vi "Get Spectrum.vi"(8 "error in (no error)":errorcluster, 10 "Channel":u8, 11 "Ocean Optics Driver in":refnum<class "Ocean Optics Driver.lvclass">) -> (0 "error out":errorcluster, 2 "Spectrum Graph":T1(graph), 3 "Ocean Optics Driver out":refnum<class "Ocean Optics Driver.lvclass">)   [LabVIEW 2016, in "Ocean Optics Driver.lvclass"]
uses:
  Ocean Optics Driver.lvclass
  <instrlib>/Ocean Optics 2000 4000/Ocean Optics 2000 4000.lvlib
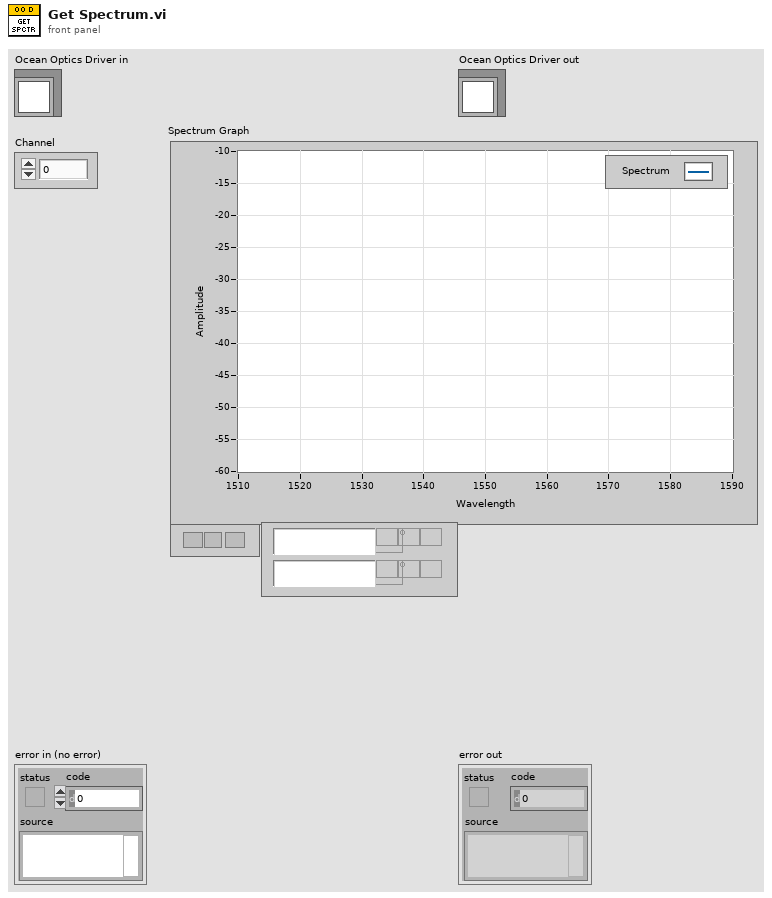
[diagram p1: front panel]
types:
  T1 = cluster{"Wavelengths":dbl[], "Spectrum by Pixel Number":dbl[]}[]
  T2 = typedef "Ocean optics configuration.ctl" = cluster{"Integration time":dbl, "Fit parameters":T3, "Fit":bool, "Auto-update params":bool, "Save spectra":bool}
  T3 = typedef "Multi-peak Parameters.ctl" = cluster{"Peaks":T4[], "Function":enum16{"Gauss", "Lorentz"}, "Window width":dbl}
  T4 = typedef "Peak Parameters.ctl" = cluster{"Amplitude":dbl, "Center":dbl, "Width":dbl}
  T5 = cluster{"Accessors:Wavelengths":dbl[], "Spectrum by Pixel Number":dbl[]}
  T6 = cluster{"Accessors:Wavelengths":dbl[], "Spectrum by Pixel Number":dbl[]}[]
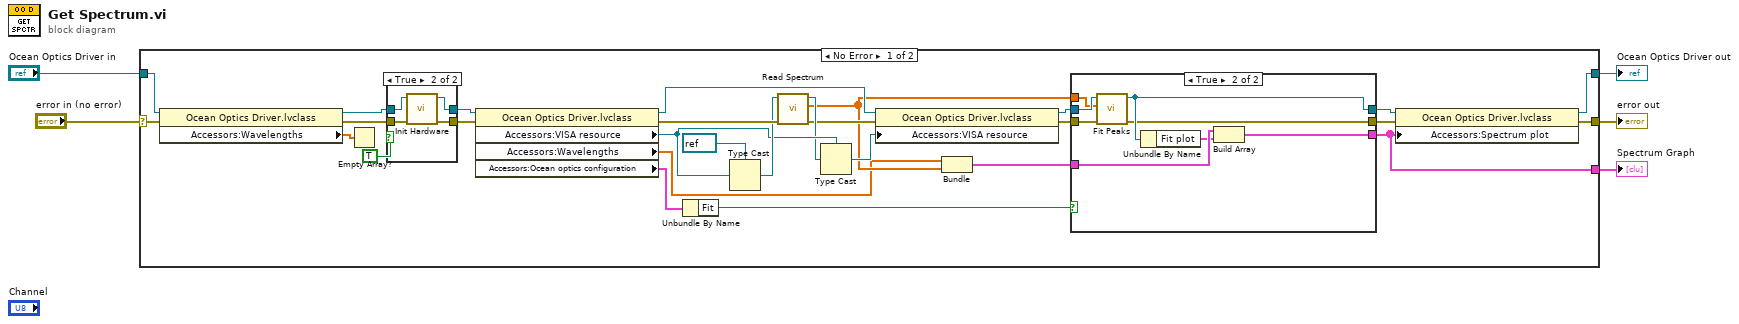
[diagram p0: block diagram]
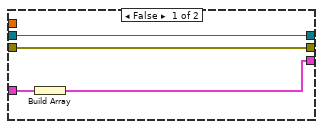
[diagram p3: hidden frame]
diagram:
  n1 = case shown="No Error" "error in (no error)" {
    selector: "error in (no error)" -> [w14 w52]
    tunnel: "Ocean Optics Driver in" -> [w12 w53]
    tunnel: [w18 w52] -> w4
    tunnel: [w16 w53] -> w3
    tunnel: [w15 _] -> w2
    frame No Error {
      n2 = property class="Ocean Optics Driver.lvclass"(reference=w12, error in=w14) -> (reference out=w10:refnum<class "Ocean Optics Driver.lvclass">, error out=w9:errorcluster, "Accessors:Wavelengths"=w11:dbl[])
      n3 = Empty Array?(array=w11) -> ()  [unwired: 1 out]
      n4 = case shown="True" TRUE {
        tunnel: w10 -> [w35 w39]
        tunnel: w9 -> [w34 w38]
        tunnel: [w35 w37] -> w8
        tunnel: [w34 w36] -> w7
        frame False {
        }
        frame True {
          n5 = call-dynamic "Init Hardware.vi"("error in (no error)"=w38, "Ocean Optics Driver in"=w39) -> ("error out"=w36:errorcluster, "Ocean Optics Driver out"=w37:refnum<class "Ocean Optics Driver.lvclass">)  [unwired: 8 in]
        }
      }
      n6 = property class="Ocean Optics Driver.lvclass"(reference=w8, error in=w7) -> (reference out=w28:refnum<class "Ocean Optics Driver.lvclass">, error out=w32:errorcluster, "Accessors:VISA resource"=w30:refnum<visa-resource-name>, "Accessors:Wavelengths"=w13:dbl[], "Accessors:Ocean optics configuration"=w25:T2)
      n7 = Unbundle By Name(w25) -> ("Fit"=w24:bool)
      n8 = Type Cast(type=refnum<visa-resource-name> refnum ("VISA resource name"), x=w30) -> (*(type *) &x=w31:refnum<visa-resource-name>)
      n9 = call <instrlib>:"Read Spectrum.vi"("error in (no error)"=w32, "VISA resource name"=w31) -> ("error out"=w26:errorcluster, "Spectrum by Pixel Number"=w21:dbl[], "VISA resource name out"=w29:refnum<visa-resource-name>)  [unwired: 6 in, 1 out]
      n10 = Type Cast(type=w30, x=w29) -> (*(type *) &x=w27:refnum<visa-resource-name>)
      n11 = property class="Ocean Optics Driver.lvclass"(reference=w28, error in=w26, "Accessors:VISA resource"=w27) -> (reference out=w23:refnum<class "Ocean Optics Driver.lvclass">, error out=w22:errorcluster)
      n12 = Bundle("Accessors:Wavelengths"=w13, "Spectrum by Pixel Number"=w21) -> (w19:T5)  [unwired: 1 out]
      n13 = case shown="True" w24 {
        tunnel: w23 -> [w41 w51]
        tunnel: w22 -> [w40 w50]
        tunnel: w21 -> [_ w49]
        tunnel: w19 -> [w43 w48]
        tunnel: [w42 w46] -> w15
        tunnel: [w41 w45] -> w17
        tunnel: [w40 w44] -> w20
        frame False {
          n14 = Build Array(w43) -> (w42:T6)
        }
        frame True {
          n15 = call-dynamic "Fit Peaks.vi"("error in (no error)"=w50, "Y"=w49, "Ocean Optics Driver in"=w51) -> ("error out"=w44:errorcluster, "Ocean Optics Driver out"=w45:refnum<class "Ocean Optics Driver.lvclass">)  [unwired: 7 in]
          n16 = Unbundle By Name(w45) -> ("Fit plot"=w47:cluster{"Array":dbl[], "Array":dbl[]})
          n17 = Build Array(w48, w47) -> (w46:cluster{"Array":dbl[], "Array":dbl[]}[])
        }
      }
      n18 = property class="Ocean Optics Driver.lvclass"(reference=w17, error in=w20, "Accessors:Spectrum plot"=w15) -> (reference out=w16:refnum<class "Ocean Optics Driver.lvclass">, error out=w18:errorcluster)
    }
    frame Error {
    }
  }
  "error out" <- w4
  "Ocean Optics Driver out" <- w3
  "Spectrum Graph" <- w2
